vi "Identify_bottle_types.vi"(11 "Array":T1(array[cluster])) -> (1 "Mixture bottles":string[](array[string]), 2 "Blank bottles":string[](array[string]), 3 "Monomolecular bottles":string[](array[string]))   [LabVIEW 2016]
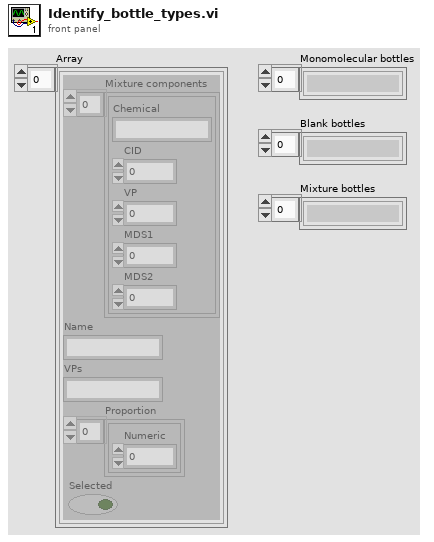
[diagram p1: front panel]
types:
  T1 = cluster{"Mixture components":cluster{"Chemical":string, "CID":i32, "VP":dbl, "MDS1":dbl, "MDS2":dbl}[], "Name":string, "VPs":string, "Proportion":cluster{"Numeric":dbl}[], "Selected":bool}[]
  T2 = cluster{"Chemical":string, "CID":i32, "VP":dbl, "MDS1":dbl, "MDS2":dbl}[]
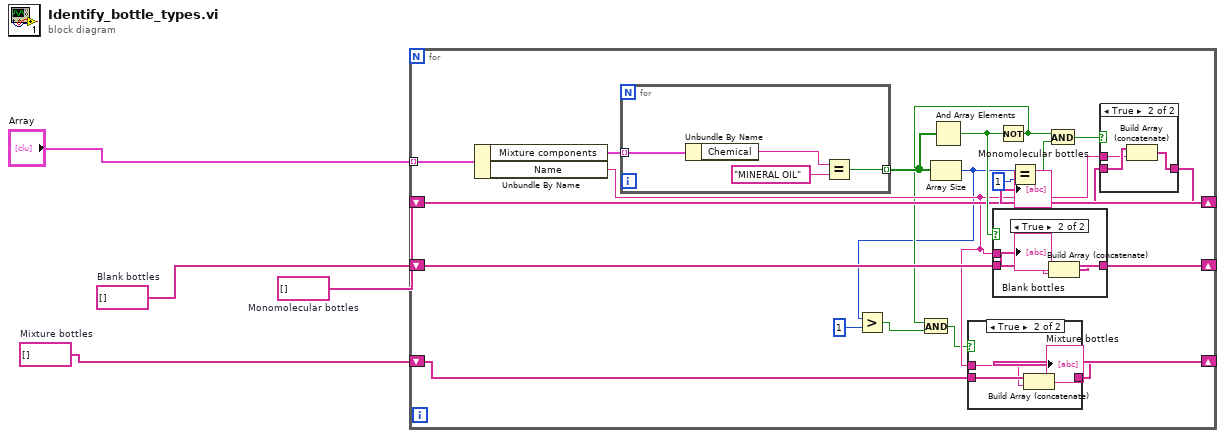
[diagram p0: block diagram]
diagram:
  w4 = string[] []  # Monomolecular bottles
  w6 = string[] []  # Mixture bottles
  w2 = string[] []  # Blank bottles
  n1 = for {
    tunnel: "Array" -> [w26] mode=indexing
    shift-right: [w23] -> w3
    shift-left: w2 -> [w24]
    shift-right: [w17] -> w5
    shift-left: w4 -> [w18]
    shift-right: [w8] -> w7
    shift-left: w6 -> [w15]
    n2 = Unbundle By Name(w26) -> ("Mixture components"=w25:T2, "Name"=w14:string)
    n3 = for {
      tunnel: w25 -> [w42] mode=indexing
      tunnel: [w39] -> w22 mode=indexing
      n4 = Unbundle By Name(w42) -> ("Chemical"=w41:string)
      n5 = Equal?(x=w41, y="MINERAL OIL") -> (x = y?=w39:bool)
    }
    n6 = Array Size(array=w22) -> (size(s)=w12:i32)
    n7 = Greater?(x=w12, y=1) -> (0:w10:bool)
    n8 = And Array Elements(Boolean array=w22) -> (logical AND=w21:bool)
    n9 = case shown="True" w21 {
      tunnel: w24 -> [w35 w38]
      tunnel: [w35 w36] -> w23
      tunnel: w14 -> [_ w37]
      frame False {
      }
      frame True {
        n10 = Build Array (concatenate)(w38, w37) -> (w36:string[])
      }
    }
    n11 = Not(x=w21) -> (.not. x?=w13:bool)
    n12 = And(x=w13, y=w10) -> (x .and. y?=w9:bool)
    n13 = case shown="True" w9 {
      tunnel: w15 -> [w27 w30]
      tunnel: [w27 w28] -> w8
      tunnel: w14 -> [_ w29]
      frame False {
      }
      frame True {
        n14 = Build Array (concatenate)(w30, w29) -> (w28:string[])
      }
    }
    n15 = Equal?(x=w12, y=1) -> (x = y?=w19:bool)
    n16 = And(x=w13, y=w19) -> (x .and. y?=w16:bool)
    n17 = case shown="True" w16 {
      tunnel: w18 -> [w31 w34]
      tunnel: [w31 w32] -> w17
      tunnel: w14 -> [_ w33]
      frame False {
      }
      frame True {
        n18 = Build Array (concatenate)(w34, w33) -> (w32:string[])
      }
    }
  }
  "Mixture bottles" <- w7
  "Monomolecular bottles" <- w5
  "Blank bottles" <- w3
